vi "Grava LOG T chips.vi"(8 "error in":errorcluster, 10 "Array ChipID+Temp":u32[](array[numeric]) format="%08x", 11 "Temperature mean":sgl) -> (0 "error out":errorcluster)   [LabVIEW 2015, in "VIPM2.lvlib"]
doc: "LOG: temperatura dels chips.\nFile path: C:\\VIP Module x2\\Files\\T chips.log\nSi no existeix l'arxiu, el crea.\nAfegeix els registres al final de l'arxiu.\nSi és 1a execució o canvi de dia, afegeix una capçalera."
uses:
  VIPM2.lvlib
panel:
  # "LOG: temperatura dels chips"
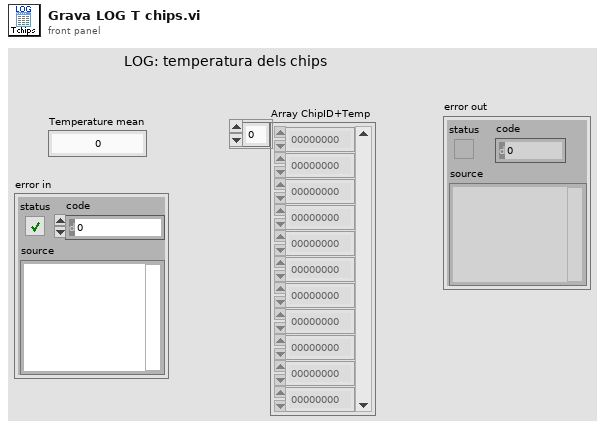
[diagram p1: front panel]
types:
  T1 = enum16{"open", "replace", "create", "open or create", "replace or create", "replace or create with confirmation"}
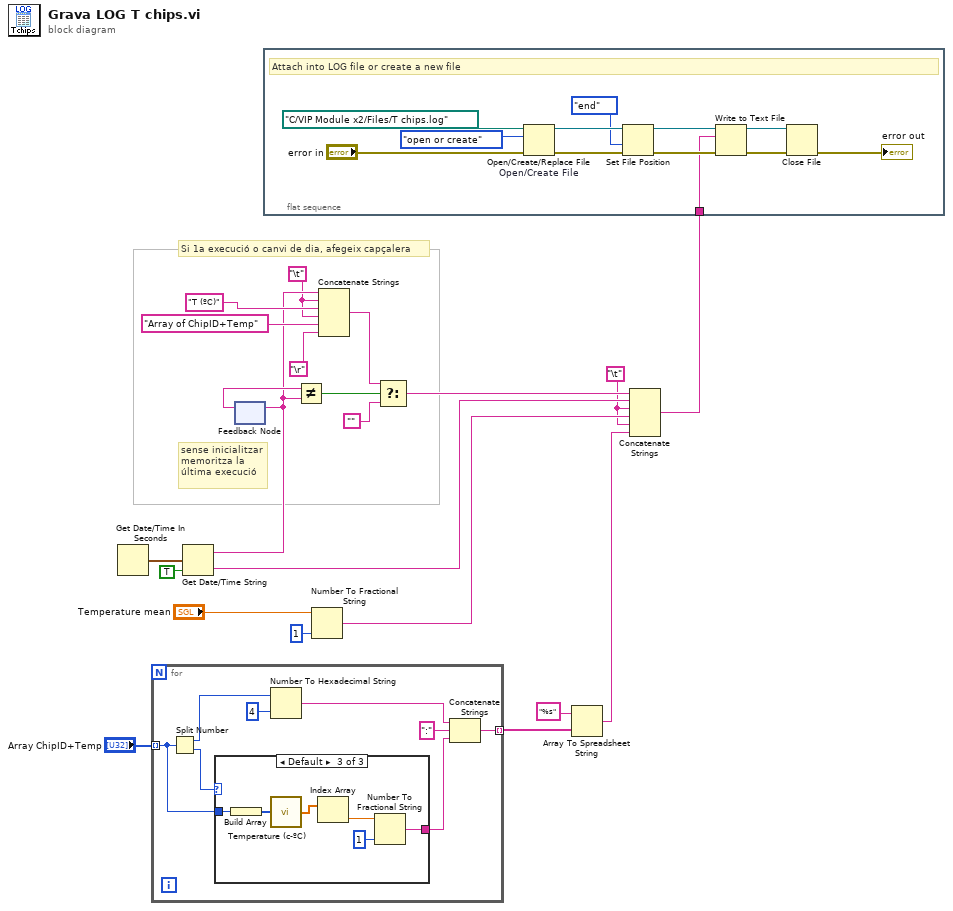
[diagram p0: block diagram]
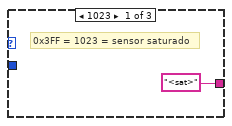
[diagram p2: hidden frame]
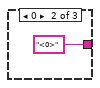
[diagram p3: hidden frame]
diagram:
  w8 = "\t"
  w7 = "\t"
  # "sense inicialitzar\nmemoritza la\núltima execució"
  # "Si 1a execució o canvi de dia, afegeix capçalera"
  n1 = Get Date/Time In Seconds() -> (seconds since 1Jan1904=w22:timestamp)
  n2 = for {
    tunnel: "Array ChipID+Temp" -> [w23] mode=indexing
    tunnel: [w25] -> w2 mode=indexing
    n3 = Split Number(x=w23) -> (hi(x)=w30:u16, lo(x)=w24:u16)
    n4 = case shown="Default" w24 {
      tunnel: ["<sat>" "<0>" w37] -> w26
      tunnel: w23 -> [_ _ w36]
      frame 1023 {
        # "0x3FF = 1023 = sensor saturado"
      }
      frame 0 {
      }
      frame Default {
        n5 = Build Array(w36) -> (w35:u32[])
        n6 = call "Temperature (c-ºC).vi"("ChipID + Tcounts"=w35) -> ("Temperatures in ºC"=w33:sgl[])  [unwired: 3 in]
        n7 = Index Array(array=w33) -> (element=w34:sgl)  [unwired: 1 in]
        n8 = Number To Fractional String(number=w34, precision (6)=i16 1) -> (F-format string=w37:string)  [unwired: 2 in]
      }
    }
    n9 = Number To Hexadecimal String(1:i16 4 ("width (-)"), 2:w30) -> (0:w28:string)
    n10 = Concatenate Strings(w28, ":" ("string"), w26) -> (w25:string)
  }
  n11 = Get Date/Time String(seconds (now)=w22, want seconds? (F)=TRUE) -> (date string=w9:string, time string=w15:string)  [unwired: 1 in]
  n12 = feedback-in #1(w9) -> ()
  n13 = feedback #1() -> (w20:string)  [unwired: 1 in]
  n14 = flat-sequence {
    tunnel: w14 -> [w41]
    frame #0 {
      # "Attach into LOG file or create a new file"
      n15 = Open/Create/Replace File "Open/Create File"(file path (use dialog)=path "C:/VIP Module x2/Files/T chips.log", error in="error in", operation (0:open)=T1."open or create") -> (refnum out=w48:refnum<file>, error out=w47:errorcluster)  [unwired: 3 in, 1 out]
      n16 = Set File Position(refnum=w48, from (0:start)=enum16{"start", "end", "current"}."end", error in=w47) -> (refnum out=w45:refnum<file>, error out=w44:errorcluster)  [unwired: 1 in]
      n17 = Write to Text File(file (use dialog)=w45, text=w41, error in=w44) -> (refnum out=w43:refnum<file>, error out=w42:errorcluster)  [unwired: 1 in, 1 out]
      n18 = Close File(refnum=w43, error in=w42) -> (error out=→"error out":errorcluster)  [unwired: 1 out]
    }
  }
  n19 = Not Equal?(x=w20, y=w9) -> (x != y?=w17:bool)
  n20 = Number To Fractional String(number="Temperature mean", precision (6)=i16 1) -> (F-format string=w12:string)  [unwired: 2 in]
  n21 = Concatenate Strings "Concatenate Strings"(w9, w8, "T (ºC)" ("string"), w8, "Array of ChipID+Temp" ("string"), "\r") -> (w18:string)
  n22 = Select(t=w18, s=w17, f="") -> (s? t:f=w16:string)
  n23 = Array To Spreadsheet String(array=w2, 3:"%s" ("format string")) -> (spreadsheet string=w5:string)  [unwired: 1 in]
  n24 = Concatenate Strings "Concatenate Strings"(w16, w15, w7, w12, w7, w5) -> (w14:string)
